vi "SetBinaryData.vi"(0 "SettingsFile in":refnum<class "SettingsFile.lvclass">, 5 "FileName":string, 7 "MD5":string, 9 "BinaryData":string, 11 "error in (no error)":errorcluster) -> (4 "SettingsFile out":refnum<class "SettingsFile.lvclass">, 6 "MD5 is same":bool, 15 "error out":errorcluster)   [LabVIEW 2018, in "SettingsFile.lvclass"]
uses:
  SettingsFile.lvclass
  SettingsFile.lvclass/SettingsFile.ctl
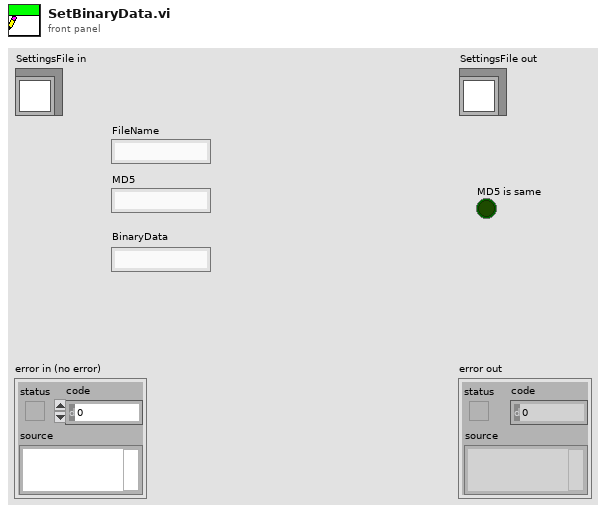
[diagram p1: front panel]
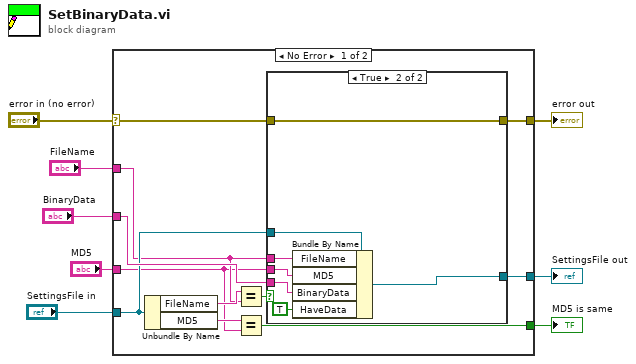
[diagram p0: block diagram]
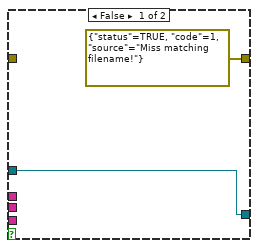
[diagram p2: hidden frame]
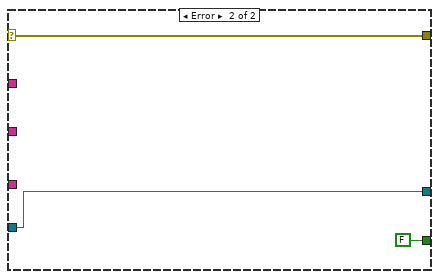
[diagram p3: hidden frame]
diagram:
  n1 = case shown="No Error" "error in (no error)" {
    selector: "error in (no error)" -> [w13 w30]
    tunnel: [w12 w30] -> w7
    tunnel: [w19 w31] -> w5
    tunnel: "SettingsFile in" -> [w17 w31]
    tunnel: "BinaryData" -> [w18 _]
    tunnel: "MD5" -> [w10 _]
    tunnel: "FileName" -> [w15 _]
    tunnel: [w9 FALSE] -> w1
    frame No Error {
      n2 = Unbundle By Name(w17) -> ("FileName"=w16:string, "MD5"=w11:string)
      n3 = Equal?(x=w16, y=w15) -> (x = y?=w14:bool)
      n4 = Equal?(x=w11, y=w10) -> (x = y?=w9:bool)
      n5 = case shown="True" w14 {
        tunnel: [w21 w28] -> w19
        tunnel: w18 -> [_ w27]
        tunnel: w10 -> [_ w26]
        tunnel: w17 -> [w21 w25]
        tunnel: w15 -> [_ w24]
        tunnel: w13 -> [_ w23]
        tunnel: [errorcluster {"status"=TRUE, "code"=1, "source"="Miss matching filename!"} ("error IO") w23] -> w12
        frame False {
        }
        frame True {
          n6 = Bundle By Name(cluster=w25, "FileName"=w24, "MD5"=w26, "BinaryData"=w27, "HaveData"=TRUE) -> (w28:refnum<class "SettingsFile.lvclass">)
        }
      }
    }
    frame Error {
    }
  }
  "error out" <- w7
  "SettingsFile out" <- w5
  "MD5 is same" <- w1
